vi "查询今日累计剂量.vi"(11 "PC个人客户端.i":refnum<class "PC个人客户端.lvclass">) -> (0 "今日数据（日期 时刻 值）":string[][](array[string]), 1 "累计剂量":string, 2 "今日日期":string, 3 "查询结果":T1)   [LabVIEW 2013, in "数据库操作.lvclass"]
uses:
  <vilib>/Utility/file.llb/Read From Spreadsheet File (string).vi
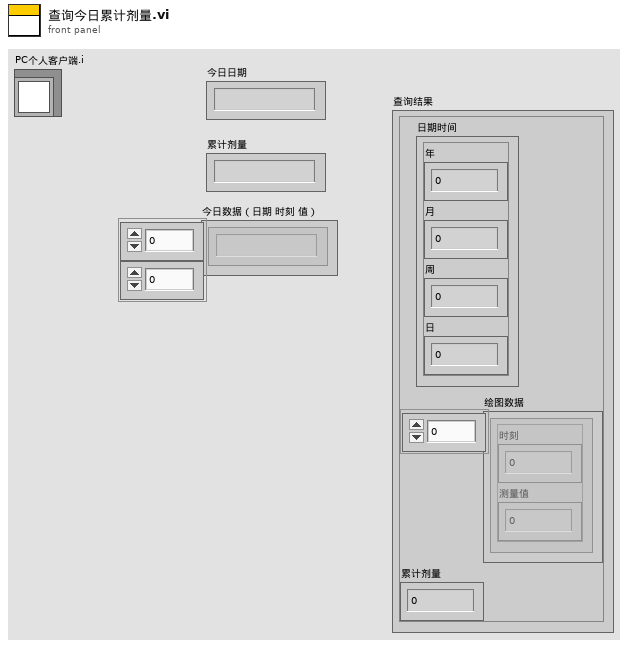
[diagram p1: front panel]
types:
  T1 = cluster{"绘图数据":cluster{"时刻":i32, "测量值":dbl}[], "累计剂量":dbl, "日期时间":cluster{"年":i32, "月":i32, "周":i32, "日":i32}}
  T2 = cluster{"用户名":string, "设备MAC":string, "设备状态":dbl, "密码":string, "职类":dbl, "姓名":string, "电话":string, "邮箱":string, "备注":string, "最后活动":string}
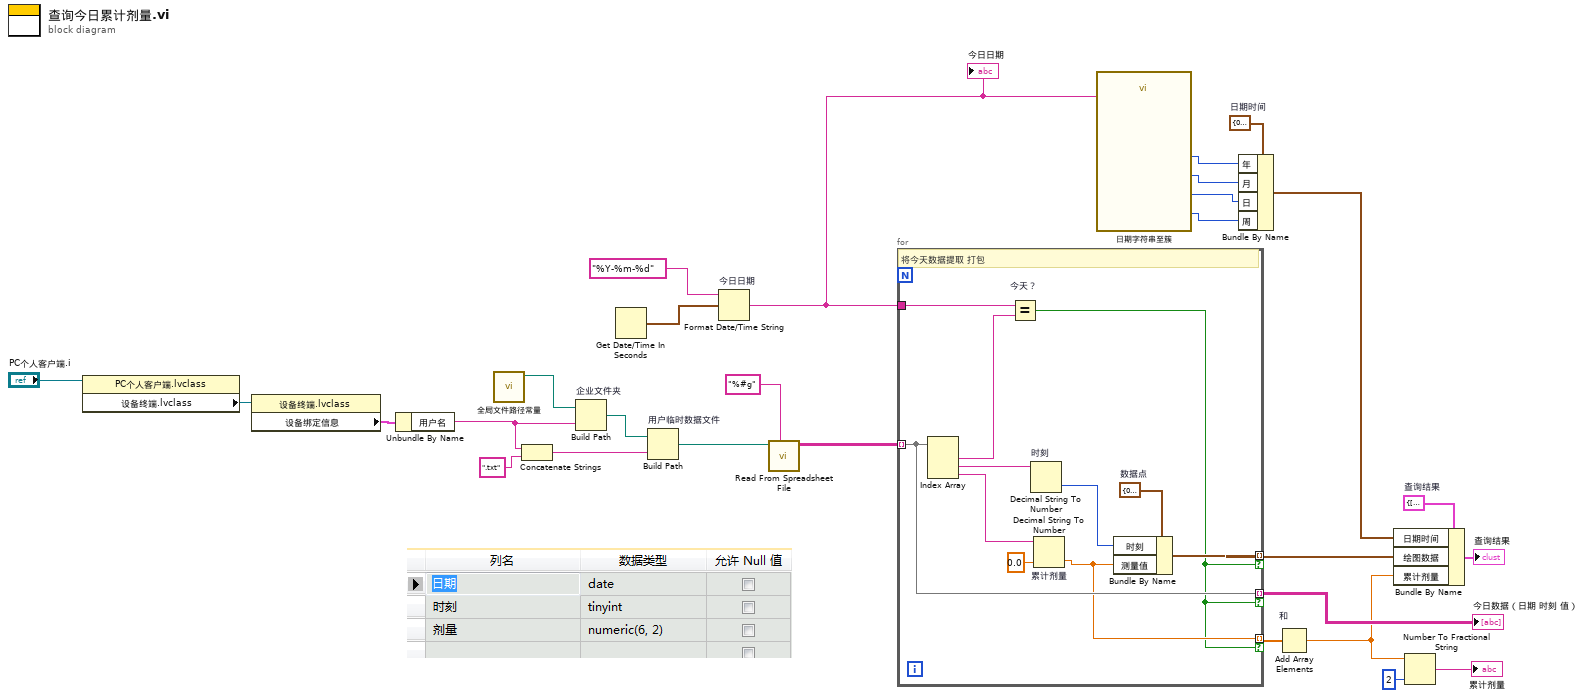
[diagram p0: block diagram]
diagram:
  w12 = cluster{"年":i32, "月":i32, "周":i32, "日":i32} {"年"=0, "月"=0, "周"=0, "日"=0}  # 日期时间
  w10 = T1 {"绘图数据"=[], "累计剂量"=0.0, "日期时间"={"年"=0, "月"=0, "周"=0, "日"=0}}  # 查询结果
  n1 = property class="PC个人客户端.lvclass"(reference="PC个人客户端.i") -> ("设备终端.lvclass"=w27:refnum<class "设备终端.lvclass">)  [unwired: 1 in, 2 out]
  n2 = property class="设备终端.lvclass"(reference=w27) -> ("设备绑定信息"=w20:T2)  [unwired: 1 in, 2 out]
  n3 = Unbundle By Name(w20) -> ("用户名"=w1:string)
  n4 = call "全局文件路径常量.vi"() -> ("用户数据库根目录"=w23:path)  [unwired: 9 in, 2 out]
  n5 = Concatenate Strings(w1, ".txt" ("字符串")) -> (w25:string)
  n6 = Build Path "企业文件夹"(base path=w23, name or relative path=w1) -> (appended path=w24:path)
  n7 = Get Date/Time In Seconds() -> (seconds since 1Jan1904=w17:timestamp)
  n8 = Build Path "用户临时数据文件"(base path=w24, name or relative path=w25) -> (appended path=w21:path)
  n9 = Format Date/Time String "今日日期"(time format string (%c)="%Y-%m-%d" ("时间格式字符串(%c)"), seconds (now)=w17) -> (date/time string=w11:string)  [unwired: 1 in]
  "今日日期" <- w11
  n10 = call-poly <vilib>:"Read From Spreadsheet File.vi"("format (%s)"="%#g", "file path (dialog if empty)"=w21) -> ("all rows"=w19:string[][])  [unwired: 5 in, 4 out]
  n11 = for {
    tunnel: w19 -> [w31] mode=indexing
    tunnel: w11 -> [w38]
    tunnel: [w32] -> w8 mode=indexing if=w29
    tunnel: [w31] -> w7 mode=indexing if=w29
    tunnel: [w30] -> w6 mode=indexing if=w29
    w34 = cluster{"时刻":i32, "测量值":dbl} {"时刻"=0, "测量值"=0.0}  # 数据点
    # "将今天数据提取 打包"
    n12 = Index Array(array=w31) -> (element #1=w39:string, element #2=w37:string, element #3=w36:string)  [unwired: 3 in]
    n13 = Equal? "今天？"(x=w38, y=w39) -> (x = y?=w29:bool)
    n14 = Decimal String To Number "时刻"(string=w37) -> (number=w33:i32)  [unwired: 2 in, 1 out]
    n15 = Decimal String To Number "累计剂量"(string=w36, default (0L)=0.0 ("默认(0 I32)")) -> (number=w30:dbl)  [unwired: 1 in, 1 out]
    n16 = Bundle By Name(cluster=w34, "时刻"=w33, "测量值"=w30) -> (w32:cluster{"时刻":i32, "测量值":dbl})
  }
  "今日数据（日期 时刻 值）" <- w7
  n17 = call "日期字符串至簇.vi"("字符串"=w11) -> ("月内周"=w16:i32, "日"=w15:i32, "月"=w14:i32, "年"=w13:i32)  [unwired: 7 in]
  n18 = Bundle By Name(cluster=w12, "年"=w13, "月"=w14, "日"=w15, "周"=w16) -> (w9:cluster{"年":i32, "月":i32, "周":i32, "日":i32})
  n19 = Add Array Elements "和"(numeric array=w6) -> (sum=w5:dbl)
  n20 = Bundle By Name(cluster=w10, "日期时间"=w9, "绘图数据"=w8, "累计剂量"=w5) -> (→"查询结果":T1)
  n21 = Number To Fractional String(number=w5, precision (6)=i16 2 ("精度(6)")) -> (F-format string=→"累计剂量":string)  [unwired: 2 in]
